vi "Set Output Level.vi"(8 "error in (no error)":errorcluster, 9 "Output Level":u32(ring)=1 items=["TTL"=1, "NIM"=2, "ECL"=3], 10 "Pulse Width":u32=2 min=2 max=255, 11 "DG Number":i32) -> (0 "error out":errorcluster)   [LabVIEW 2009]
doc: "long Set_OutputLevel(unsigned long OutputLevel, unsigned long PulseWidth, long DG_Number);"
uses:
  DelayGenerator.dll
panel:
  # "NOTICE -- YOU MUST LEAVE THIS NOTICE IN PLACE.  PER THE TERMS OF THE LICENSE BELOW, YOU MAY SUBLICENSE THIS SOFTWARE \nIN ANY WAY THAT DOES NOT CONFLICT WITH THIS LICENSE.\n\n### BSD License (http://www.opensource.org/licenses/bsd-license.php) Begin ###\n \nCopyright (c) 2011, Applied Energetics, http://www.appliedenergetics.com,\n                               Richard Schwerdtfeger, <rschwerdtfeger@appliedenergetics.com>\n\nAll rights reserved.\n\nRedistribution and use in source and binary forms, with or without modification, are permitted provided that the \nfollowing conditions are met:\n\n    * Redistributions of source code must retain the above copyright notice, this list of conditions and the following disclaimer.\n    * Redistributions in binary form must reproduce the above copyright notice, this list of conditions and the following disclaimer \n       in the documentation and/or other materials provided with the distribution.\n    * Neither the name of Richard Schwerdtfeger, Applied Energetics, Inc., nor the names of its contributors may be used to \n       endorse or promote products derived from this software without specific prior written permission.\n\nTHIS SOFTWARE IS PROVIDED BY THE COPYRIGHT HOLDERS AND CONTRIBUTORS \"AS IS\" AND ANY EXPRESS OR IMPLIED WARRANTIES, \nINCLUDING, BUT NOT LIMITED TO, THE IMPLIED WARRANTIES OF MERCHANTABILITY AND FITNESS FOR A PARTICULAR PURPOSE ARE \nDISCLAIMED. IN NO EVENT SHALL THE COPYRIGHT OWNER OR CONTRIBUTORS BE LIABLE FOR ANY DIRECT, INDIRECT, INCIDENTAL,\n SPECIAL, EXEMPLARY, OR CONSEQUENTIAL DAMAGES (INCLUDING, BUT NOT LIMITED TO, PROCUREMENT OF SUBSTITUTE GOODS OR \nSERVICES; LOSS OF USE, DATA, OR PROFITS; OR BUSINESS INTERRUPTION) HOWEVER CAUSED AND ON ANY THEORY OF LIABILITY, \nWHETHER IN CONTRACT, STRICT LIABILITY, OR TORT (INCLUDING NEGLIGENCE OR OTHERWISE) ARISING IN ANY WAY OUT OF THE USE \nOF THIS SOFTWARE, EVEN IF ADVISED OF THE POSSIBILITY OF SUCH DAMAGE.\n\n### BSD License End ###"
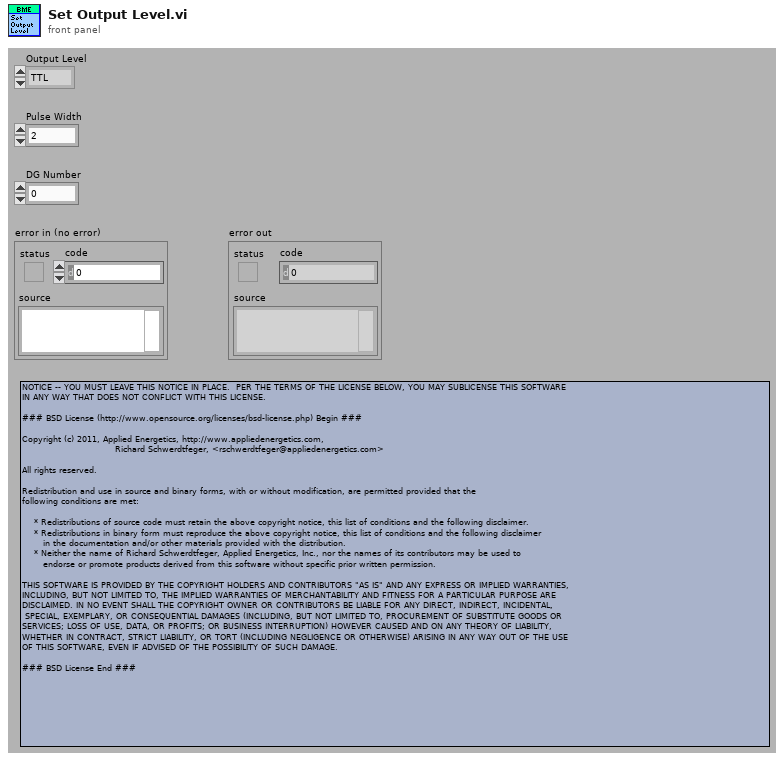
[diagram p1: front panel]
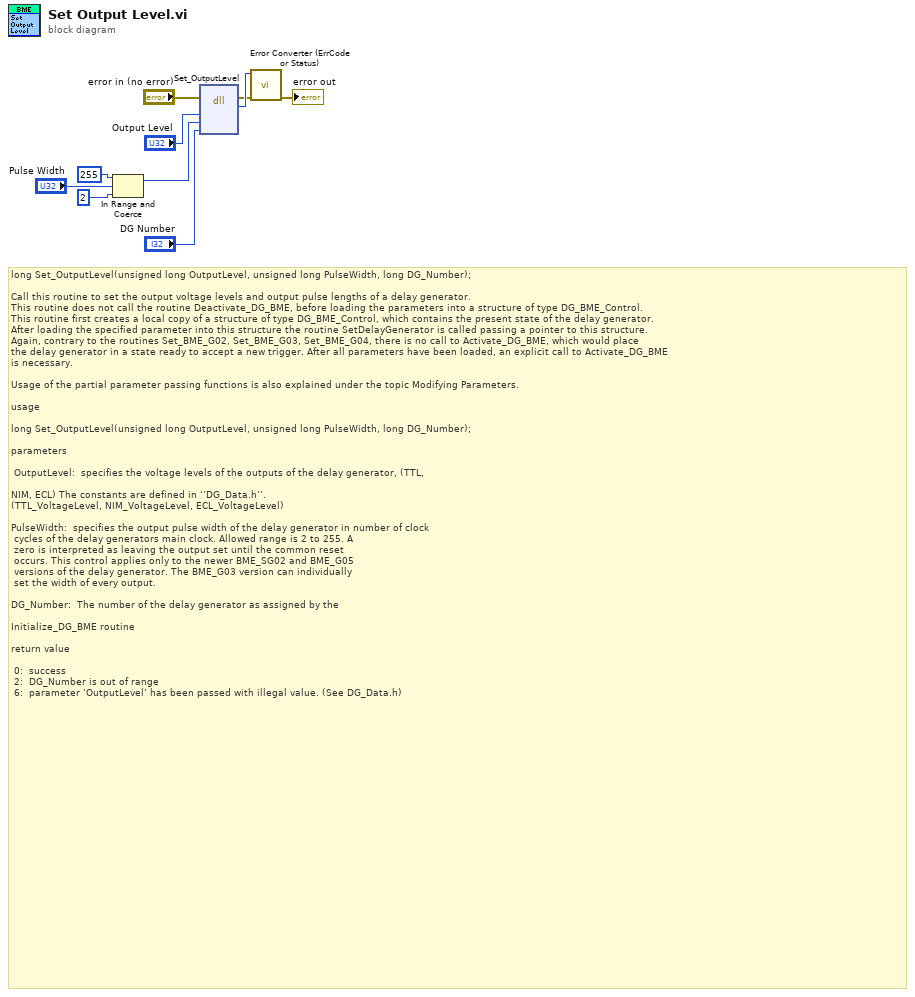
[diagram p0: block diagram]
diagram:
  # "long Set_OutputLevel(unsigned long OutputLevel, unsigned long PulseWidth, long DG_Number);\n\nCall this routine to set the output voltage levels and output pulse lengths of a delay generator. \nThis routine does not call the routine Deactivate_DG_BME, before loading the parameters into a structure of type DG_BME_Control. \nThis routine first creates a local copy of a structure of type DG_BME_Control, which contains the present state of the delay generator. \nAfter loading the specified parameter into this structure the routine SetDelayGenerator is called passing a pointer to this structure. \nAgain, contrary to the routines Set_BME_G02, Set_BME_G03, Set_BME_G04, there is no call to Activate_DG_BME, which would place \nthe delay generator in a state ready to accept a new trigger. After all parameters have been loaded, an explicit call to Activate_DG_BME \nis necessary.\n\nUsage of the partial parameter passing functions is also explained under the topic Modifying Parameters.\n\nusage\n\nlong Set_OutputLevel(unsigned long OutputLevel, unsigned long PulseWidth, long DG_Number);\n\nparameters\n\n\tOutputLevel:\t\tspecifies the voltage levels of the outputs of the delay generator, (TTL,\n\nNIM, ECL) The constants are defined in ‘’DG_Data.h’’.\n(TTL_VoltageLevel, NIM_VoltageLevel, ECL_VoltageLevel)\n\nPulseWidth:\t\tspecifies the output pulse width of the delay generator in number of clock\n cycles of the delay generators main clock. Allowed range is 2 to 255. A\n zero is interpreted as leaving the output set until the common reset \n occurs. This control applies only to the newer BME_SG02 and BME_G05\n versions of the delay generator. The BME_G03 version can individually\n set the width of every output.\n\nDG_Number:\t\tThe number of the delay generator as assigned by the\n\nInitialize_DG_BME routine\n\nreturn value\n\n\t0:  success\n\t2:  DG_Number is out of range\n\t6:  parameter ‘OutputLevel’ has been passed with illegal value. (See DG_Data.h)"
  n1 = In Range and Coerce(upper limit=u32 255, x="Pulse Width", lower limit=u32 2) -> (coerced(x)=w4:u32)  [unwired: 1 out]
  n2 = dll-call lib="C:/Dokumente und Einstellungen/A2.5/Desktop/BME_SW Stand 201203-26/LabView_SG08p/BME Delay Generator/DelayGenerator.*" fn="Set_OutputLevel"(error in="error in (no error)", "OutputLevel"="Output Level", "PulseWidth"=w4, "DG_Number"="DG Number") -> (error out=w6:errorcluster, w10:i32)  [unwired: 5 in, 1 out]
  n3 = call "Error Converter (ErrCode or Status).vi"("error in (no error)"=w6, "error code"=w10) -> ("error out"=→"error out":errorcluster)  [unwired: 9 out]
